vi "写 M0-M31.vi"(7 "Old VAL":bool[](array[boolean]), 8 "错误输入（无错误）":errorcluster, 10 "索引":i32, 11 "VISA资源名称":refnum<visa-resource-name>="COM2") -> (0 "错误输出":errorcluster)   [LabVIEW 2014]
uses:
  <vilib>/Instr/_visa.llb/VISA Configure Serial Port (Instr).vi
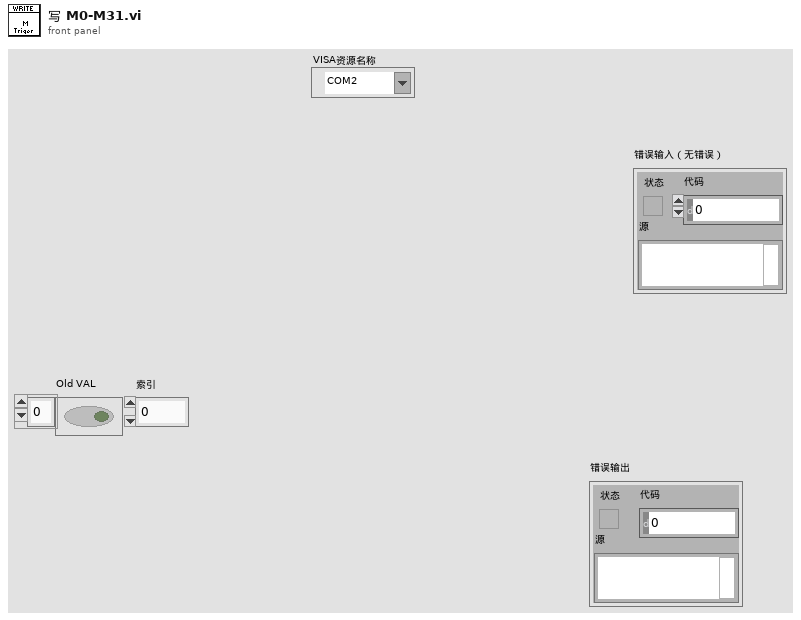
[diagram p1: front panel]
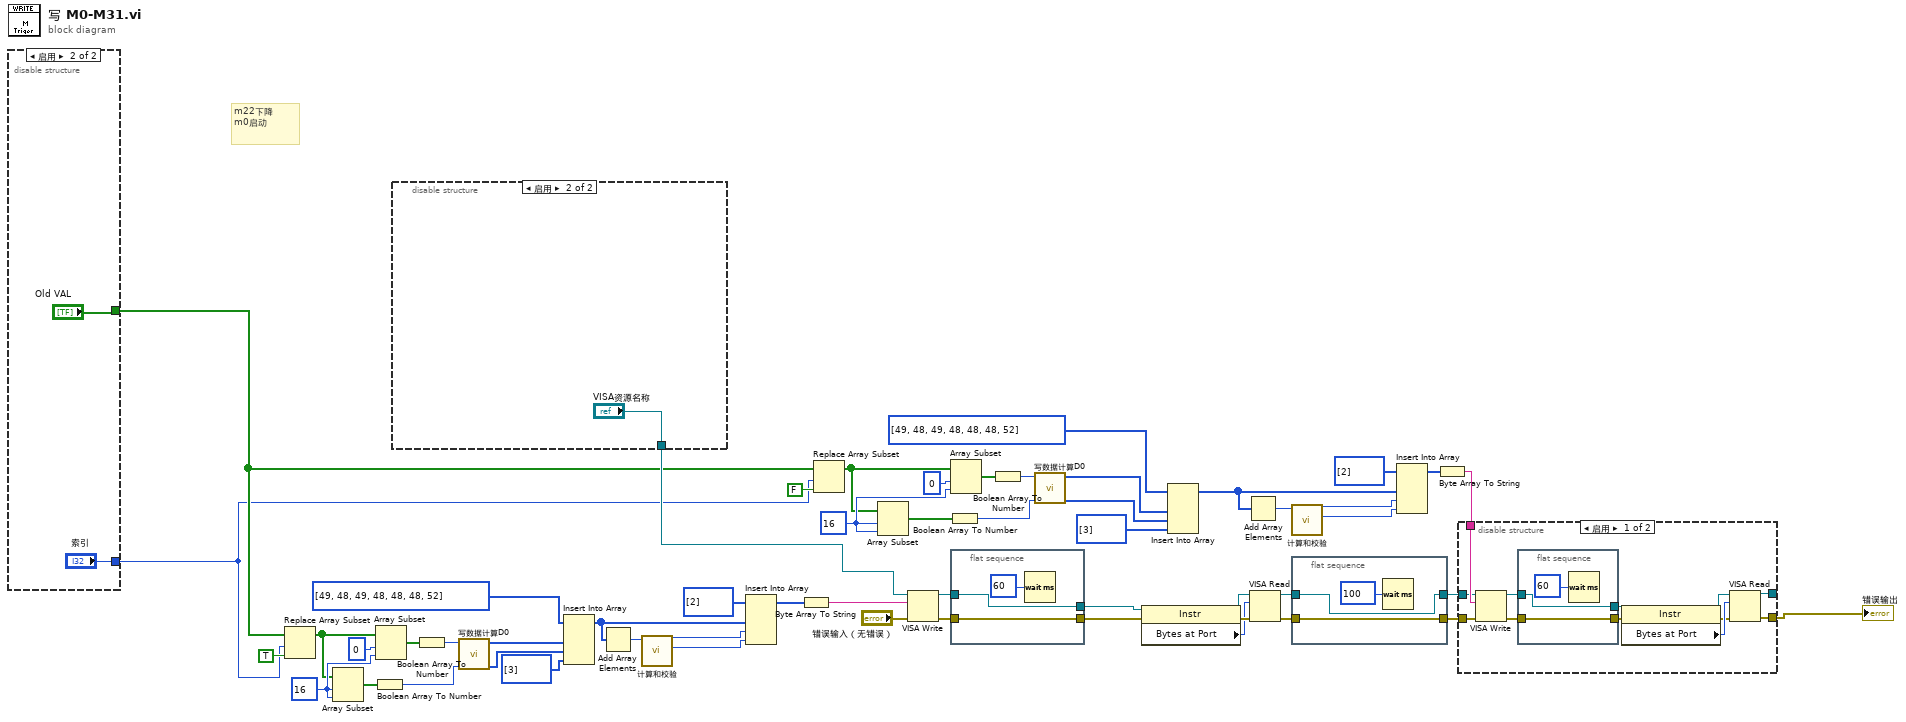
[diagram p0: block diagram]
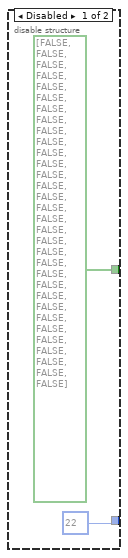
[diagram p2: hidden frame]
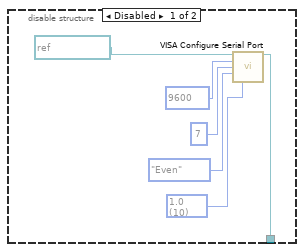
[diagram p3: hidden frame]
diagram:
  w26 = 16 ("长度")
  w32 = 16 ("长度")
  # "m22下降\nm0启动"
  n1 = disable-structure shown="启用" {
    disable-tunnel: [bool[] [FALSE, FALSE, FALSE, FALSE, FALSE, FALSE, FALSE, FALSE, FALSE, FALSE, FALSE, FALSE, FALSE, FALSE, FALSE, FALSE, FALSE, FALSE, FALSE, FALSE, FALSE, FALSE, FALSE, FALSE, FALSE, FALSE, FALSE, FALSE, FALSE, FALSE, FALSE, FALSE] ("M 2") "Old VAL"] -> w3
    disable-tunnel: [22 ("索引") "索引"] -> w2
    frame Disabled {
    }
    frame Enabled {
    }
  }
  n2 = Replace Array Subset(array=w3, new element=TRUE ("Val"), index=w2) -> (w31:bool[])
  n3 = Array Subset(array=w31, index=w32, length=w32) -> (w29:bool[])
  n4 = Boolean Array To Number(Boolean array=w29) -> (number=w34:u32)
  n5 = Array Subset(array=w31, index=0 ("索引"), length=w32) -> (w30:bool[])
  n6 = disable-structure shown="启用" {
    disable-tunnel: [w59 "VISA资源名称"] -> w4
    frame Disabled {
      w64 = u16 10 items=["1.0"=10, "1.5"=15, "2.0"=20] ("停止位")
      n7 = call-poly "VISA Configure Serial Port"("VISA resource name"=refnum<visa-resource-name> "COM2" ("VISA资源名称"), "baud rate (9600)"=u32 9600 ("波特率"), "data bits (8)"=u16 7 ("数据位"), "parity (0:none)"=enum16{"None", "Odd", "Even", "Mark", "Space"}."Even" ("校验位"), "stop bits (10: 1 bit)"=w64) -> ("VISA resource name out"=w59:refnum<visa-resource-name>)  [unwired: 9 in, 1 out]
    }
    frame Enabled {
    }
  }
  n8 = Boolean Array To Number(Boolean array=w30) -> (number=w35:u32)
  n9 = call "写数据计算D0.vi"("D0 2"=w34, "D0"=w35) -> ("数组 2"=w36:u32[], "数组"=w43:u32[])  [unwired: 8 in]
  n10 = Insert Into Array(array=u16[] [49, 48, 49, 48, 48, 48, 52], new element #1=w43, new element #2=w36, new element #3=u16[] [3]) -> (w42:u16[])  [unwired: 1 in]
  n11 = Add Array Elements(numeric array=w42) -> (sum=w39:u16)
  n12 = call "计算和校验.vi"("和"=w39) -> ("底"=w40:u32, "高"=w41:u32)  [unwired: 9 in]
  n13 = Insert Into Array(array=u16[] [2], new element #1=w42, new element #2=w41, new element #3=w40) -> (w45:u16[])  [unwired: 1 in]
  n14 = Byte Array To String(unsigned byte array=w45) -> (string=w52:string)
  n15 = Replace Array Subset(array=w3, new element=FALSE, index=w2) -> (w5:bool[])
  n16 = Array Subset(array=w5, index=w26, length=w26) -> (w28:bool[])
  n17 = VISA Write(VISA resource name=w4, write buffer=w52, error in (no error)="错误输入（无错误）") -> (VISA resource name out=w53:refnum<visa-resource-name>, error out=w54:errorcluster)  [unwired: 1 out]
  n18 = Boolean Array To Number(Boolean array=w28) -> (number=w24:u32)
  n19 = Array Subset(array=w5, index=0 ("索引"), length=w26) -> (w27:bool[])
  n20 = flat-sequence {
    tunnel: w54 -> [w68]
    tunnel: [w68] -> w47
    tunnel: w53 -> [w67]
    tunnel: [w67] -> w48
    frame #0 {
      n21 = Wait (ms)(milliseconds to wait=u32 60 ("等待时间（毫秒）")) -> ()  [unwired: 1 out]
    }
  }
  n22 = Boolean Array To Number(Boolean array=w27) -> (number=w23:u32)
  n23 = call "写数据计算D0.vi"("D0 2"=w24, "D0"=w23) -> ("数组 2"=w22:u32[], "数组"=w16:u32[])  [unwired: 8 in]
  n24 = property class="Instr"(reference=w48, error in=w47) -> (reference out=w51:refnum<visa-resource-name>, error out=w50:errorcluster, "Bytes at Port"=w49:u32)
  n25 = Insert Into Array(array=u16[] [49, 48, 49, 48, 48, 48, 52], new element #1=w16, new element #2=w22, new element #3=u16[] [3]) -> (w17:u16[])  [unwired: 1 in]
  n26 = Add Array Elements(numeric array=w17) -> (sum=w20:u16)
  n27 = VISA Read(VISA resource name=w51, byte count=w49, error in (no error)=w50) -> (VISA resource name out=w11:refnum<visa-resource-name>, error out=w10:errorcluster)  [unwired: 2 out]
  n28 = call "计算和校验.vi"("和"=w20) -> ("底"=w19:u32, "高"=w18:u32)  [unwired: 9 in]
  n29 = flat-sequence {
    tunnel: w11 -> [w70]
    tunnel: w10 -> [w69]
    tunnel: [w70] -> w9
    tunnel: [w69] -> w8
    frame #0 {
      n30 = Wait (ms)(milliseconds to wait=u32 100 ("等待时间（毫秒）")) -> ()  [unwired: 1 out]
    }
  }
  n31 = Insert Into Array(array=u16[] [2], new element #1=w17, new element #2=w18, new element #3=w19) -> (w14:u16[])  [unwired: 1 in]
  n32 = Byte Array To String(unsigned byte array=w14) -> (string=w12:string)
  n33 = disable-structure shown="启用" {
    disable-tunnel: w12 -> [w76 _]
    disable-tunnel: w9 -> [w75 w88]
    disable-tunnel: w8 -> [w74 w87]
    disable-tunnel: [w73 w88] -> _
    disable-tunnel: [w72 w87] -> w1
    frame Enabled {
      n34 = VISA Write(VISA resource name=w75, write buffer=w76, error in (no error)=w74) -> (VISA resource name out=w78:refnum<visa-resource-name>, error out=w77:errorcluster)  [unwired: 1 out]
      n35 = flat-sequence {
        tunnel: w77 -> [w86]
        tunnel: [w86] -> w83
        tunnel: w78 -> [w85]
        tunnel: [w85] -> w82
        frame #0 {
          n36 = Wait (ms)(milliseconds to wait=u32 60 ("等待时间（毫秒）")) -> ()  [unwired: 1 out]
        }
      }
      n37 = property class="Instr"(reference=w82, error in=w83) -> (reference out=w79:refnum<visa-resource-name>, error out=w80:errorcluster, "Bytes at Port"=w81:u32)
      n38 = VISA Read(VISA resource name=w79, byte count=w81, error in (no error)=w80) -> (VISA resource name out=w73:refnum<visa-resource-name>, error out=w72:errorcluster)  [unwired: 2 out]
    }
    frame Disabled {
    }
  }
  "错误输出" <- w1
